vi "Format Log.vi"(7 "Show Timestamps":bool, 8 "error in (no error)":errorcluster, 11 "LV Chat Client in":refnum<class "LV Chat Client.lvclass">) -> (0 "error out":errorcluster, 2 "Log":string, 3 "LV Chat Client out":refnum<class "LV Chat Client.lvclass">)   [LabVIEW 2020, in "LV Chat Client.lvclass"]
uses:
  LV Chat Client.lvclass
  LV Chat Client.lvclass/LV Chat Client.ctl
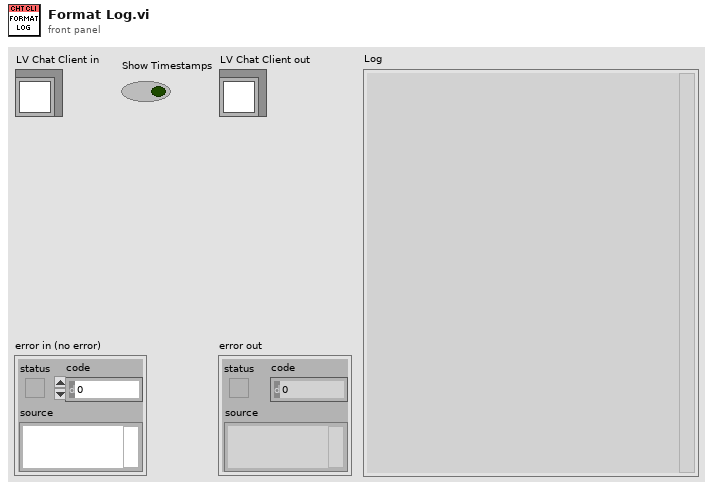
[diagram p1: front panel]
types:
  T1 = typedef "Message.ctl" = cluster{"From":string, "Time":dbl, "Message":string}
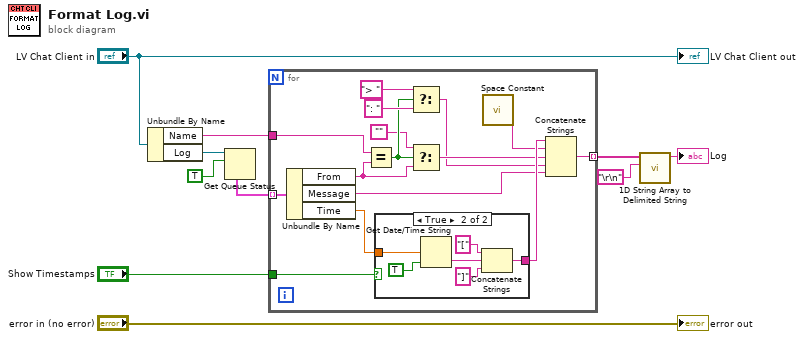
[diagram p0: block diagram]
diagram:
  n1 = Unbundle By Name("LV Chat Client in") -> ("Name"=w5:string, "Log"=w8:refnum<queue>)
  n2 = Get Queue Status(queue=w8, return elements? (F)=TRUE) -> (elements=w6:T1[])  [unwired: 1 in, 7 out]
  n3 = for {
    tunnel: w6 -> [w25] mode=indexing
    tunnel: w5 -> [w16]
    tunnel: "Show Timestamps" -> [w20]
    tunnel: [w12] -> w3 mode=indexing
    n4 = Unbundle By Name(w25) -> ("From"=w15:string, "Message"=w13:string, "Time"=w21:dbl)
    n5 = Equal?(x=w16, y=w15) -> (x = y?=w22:bool)
    n6 = case shown="True" w20 {
      tunnel: w21 -> [_ w31]
      tunnel: [_ w26] -> w19
      frame False {
      }
      frame True {
        n7 = Get Date/Time String(seconds (now)=w31, want seconds? (F)=TRUE) -> (time string=w29:string)  [unwired: 1 in, 1 out]
        n8 = Concatenate Strings("[" ("string"), w29, "]" ("string")) -> (w26:string)
      }
    }
    n9 = Select(t="> ", s=w22, f=": ") -> (s? t:f=w14:string)
    n10 = Select(t="", s=w22, f=w15) -> (s? t:f=w17:string)
    n11 = call <vilib>:"Space Constant.vi"() -> ("String"=w18:string)
    n12 = Concatenate Strings(w19, w18, w17, w14, w13) -> (w12:string)
  }
  n13 = call <vilib>:"1D String Array to Delimited String.vi"("delimiter"="\r\n", "string array"=w3) -> ("delimited string"=→"Log":string)  [unwired: 9 in]
  "error out" <- "error in (no error)"
  "LV Chat Client out" <- "LV Chat Client in"
